vi "AO voice coil and DO camera synchronization.vi"() -> ()   [LabVIEW 2020]
uses:
  <vilib>/DAQmx/write.llb/DAQmx Write (Analog Wfm 1Chan NSamp).vi
  <vilib>/DAQmx/create/channels.llb/DAQmx Create Channel (AO-Voltage-Basic).vi
  <vilib>/DAQmx/configure/timing.llb/DAQmx Timing (Sample Clock).vi
  <vilib>/DAQmx/configure/trigger.llb/DAQmx Start Trigger (Digital Edge).vi
  <vilib>/DAQmx/create/channels.llb/DAQmx Create Channel (CO-Pulse Generation-Frequency).vi
  <vilib>/DAQmx/configure/timing.llb/DAQmx Timing (Implicit).vi
  <vilib>/DAQmx/miscellaneous.llb/DAQmx Fill In Error Info.vi
  <vilib>/measure/NI_MABase.lvlib
  <resource>/objmgr/daqmx.rc
panel:
  in  "offset":dbl format="%.2p"
  out "Waveform Graph":waveform(dbl)(graph)
  in  "phase":dbl format="%.2p"
  in  "stop":bool
  in  "amplitude":dbl=1.0 format="%.2p"
  # "Voltage=250mv\nPhase=216"
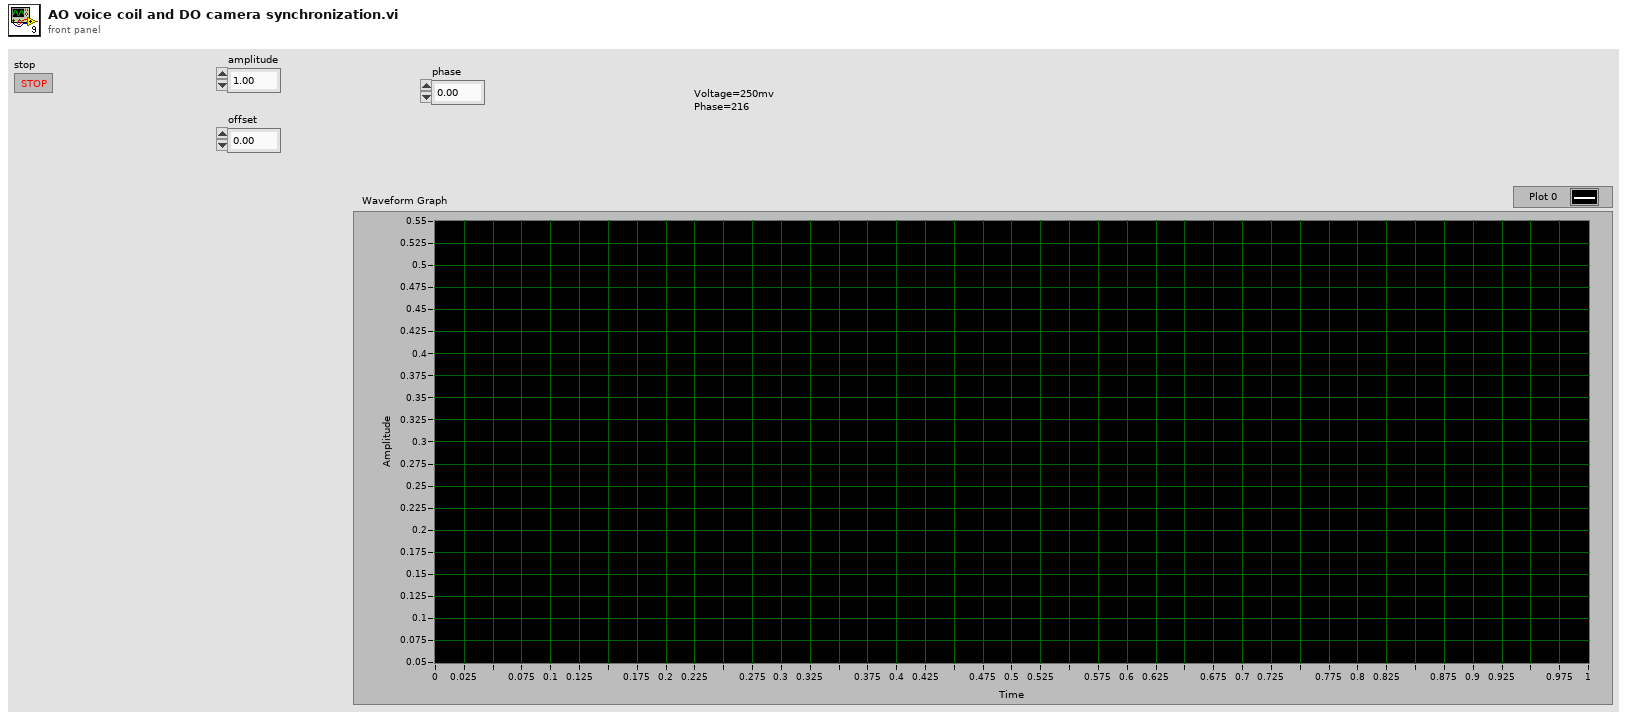
[diagram p1: front panel]
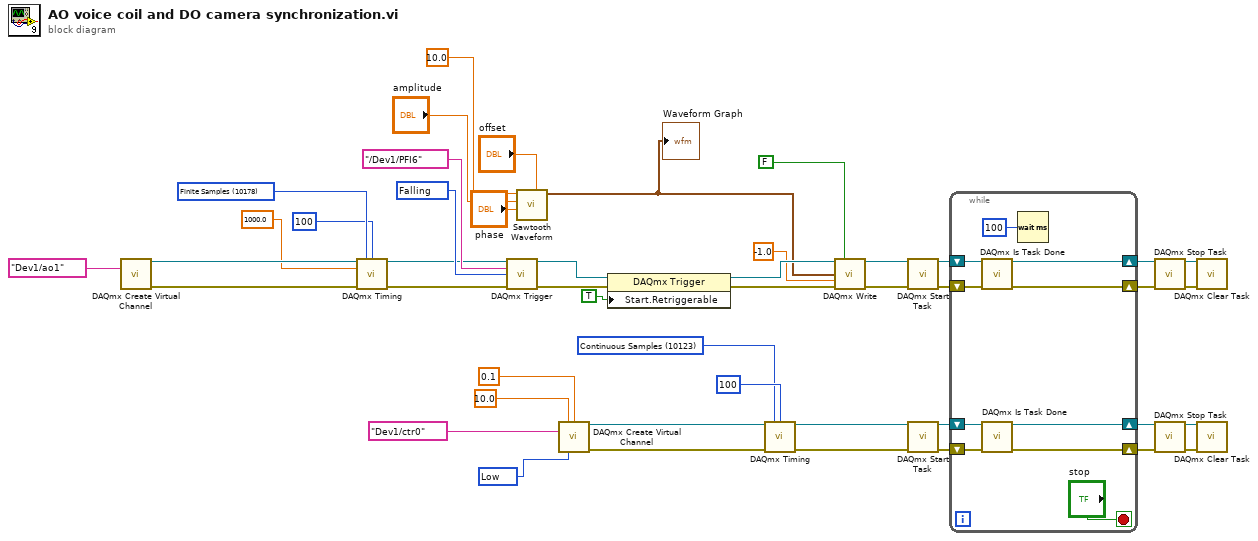
[diagram p0: block diagram]
diagram:
  w7 = 10214 items=["High"=10192, "Low"=10214] ("idle state")
  w9 = 10123 items=["Finite Samples"=10178, "Continuous Samples"=10123, "Hardware Timed Single Point"=12522] ("sample mode")
  w31 = 10178 items=["Finite Samples"=10178, "Continuous Samples"=10123, "Hardware Timed Single Point"=12522] ("sample mode")
  w33 = 10171 items=["Rising"=10280, "Falling"=10171] ("edge")
  n1 = call-poly <vilib>:"DAQmx Create Virtual Channel.vi"("physical channels"=tag "Dev1/ao1") -> ("task out"=w35:refnum<k21>, "error out"=w34:errorcluster)  [unwired: 13 in]
  n2 = call-poly <vilib>:"DAQmx Timing.vi"("task/channels in"=w35, "sample mode"=w31, "samples per channel"=100, "rate"=1000.0, "error in"=w34) -> ("task out"=w13:refnum<k21>, "error out"=w12:errorcluster)  [unwired: 9 in]
  n3 = call-poly <vilib>:"DAQmx Trigger.vi"("task/channels in"=w13, "source"=tag "/Dev1/PFI6", "edge"=w33, "error in"=w12) -> ("task out"=w19:refnum<k21>, "error out"=w32:errorcluster)  [unwired: 10 in]
  n4 = call <vilib>:"Sawtooth Waveform.vi"("offset"="offset", "phase"="phase", "amplitude"="amplitude", "frequency"=10.0) -> ("signal out"=w2:waveform(dbl))  [unwired: 6 in, 1 out]
  "Waveform Graph" <- w2
  n5 = call-poly <vilib>:"DAQmx Create Virtual Channel.vi"("frequency"=10.0, "duty cycle"=0.1, "counter"=tag "Dev1/ctr0", "idle state"=w7) -> ("task out"=w16:refnum<k21>, "error out"=w15:errorcluster)  [unwired: 10 in]
  n6 = property class="DAQmx Trigger"(reference=w19, error in=w32, "Start.Retriggerable"=TRUE) -> (reference out=w29:refnum<k21>, error out=w28:errorcluster)
  n7 = call-poly <vilib>:"DAQmx Timing.vi"("task/channels in"=w16, "sample mode"=w9, "samples per channel"=100, "error in"=w15) -> ("task out"=w5:refnum<k21>, "error out"=w4:errorcluster)  [unwired: 10 in]
  n8 = call-poly <vilib>:"DAQmx Write.vi"("task/channels in"=w29, "auto start"=FALSE, "data"=w2, "timeout"=-1.0, "error in"=w28) -> ("task out"=w24:refnum<k21>, "error out"=w25:errorcluster)  [unwired: 8 in, 1 out]
  n9 = call <vilib>:"DAQmx Start Task.vi"("task/channels in"=w24, "error in"=w25) -> ("task out"=w23:refnum<k21>, "error out"=w17:errorcluster)  [unwired: 12 in]
  n10 = call <vilib>:"DAQmx Start Task.vi"("task/channels in"=w5, "error in"=w4) -> ("task out"=w27:refnum<k21>, "error out"=w26:errorcluster)  [unwired: 12 in]
  n11 = while {
    shift-right: [w51] -> w38
    shift-left: w23 -> [w48]
    shift-right: [w54] -> w44
    shift-left: w27 -> [w56]
    shift-right: [w53] -> w42
    shift-left: w26 -> [w55]
    shift-right: [w52] -> w40
    shift-left: w17 -> [w47]
    stop <- "stop" stop-if-true
    n12 = call <vilib>:"DAQmx Is Task Done.vi"("task/channels in"=w48, "error in"=w47) -> ("task out"=w51:refnum<k21>, "error out"=w52:errorcluster)  [unwired: 11 in, 1 out]
    n13 = call <vilib>:"DAQmx Is Task Done.vi"("task/channels in"=w56, "error in"=w55) -> ("task out"=w54:refnum<k21>, "error out"=w53:errorcluster)  [unwired: 11 in, 1 out]
    n14 = Wait (ms)(milliseconds to wait=u32 100) -> ()  [unwired: 1 out]
  }
  n15 = call <vilib>:"DAQmx Stop Task.vi"("task/channels in"=w38, "error in"=w40) -> ("task out"=w37:refnum<k21>, "error out"=w39:errorcluster)  [unwired: 12 in]
  n16 = call <vilib>:"DAQmx Stop Task.vi"("task/channels in"=w44, "error in"=w42) -> ("task out"=w43:refnum<k21>, "error out"=w41:errorcluster)  [unwired: 12 in]
  n17 = call <vilib>:"DAQmx Clear Task.vi"("task in"=w37, "error in"=w39) -> ()  [unwired: 13 in, 1 out]
  n18 = call <vilib>:"DAQmx Clear Task.vi"("task in"=w43, "error in"=w41) -> ()  [unwired: 13 in, 1 out]
